vi "IsMaster.vi"(8 "error in (no error)":errorcluster, 11 "ELAN Master in":refnum<class "ELAN Master.lvclass">) -> (0 "error out":errorcluster, 2 "isMaster":bool, 3 "ELAN Master out":refnum<class "ELAN Master.lvclass">)   [LabVIEW 2021, in "ELAN Master.lvclass"]
uses:
  ELAN Master.lvclass
  ELAN Master.lvclass/ELAN Master.ctl
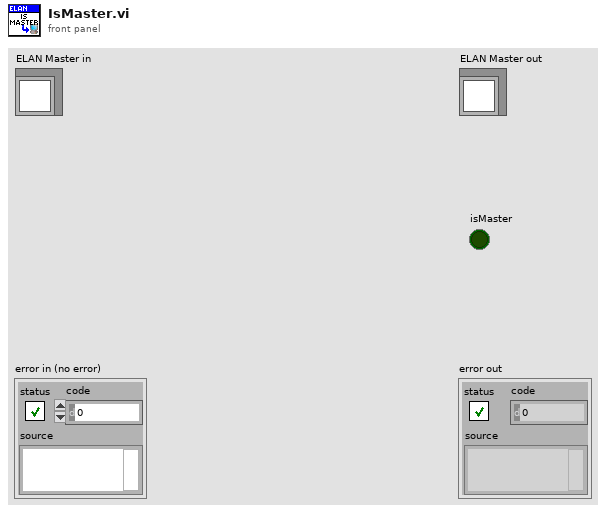
[diagram p1: front panel]
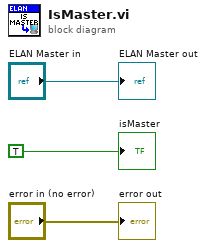
[diagram p0: block diagram]
diagram:
  "error out" <- "error in (no error)"
  "ELAN Master out" <- "ELAN Master in"
  "isMaster" <- TRUE ("isMaster")
